vi "Read I64.vi"(7 "length":u16, 8 "error in (no error)":errorcluster, 9 "Start address":string, 10 "Read Type":variant, 11 "MelsecTCP in":refnum<class "Abs Controler.lvclass">) -> (0 "error out":errorcluster, 2 "Data":variant, 3 "MelsecTCP out":refnum<class "Abs Controler.lvclass">)   [LabVIEW 2020, in "HslCommunication.lvlib" / "Abs Controler.lvclass"]
uses:
  Abs Controler.lvclass
  E:/Git/Libraries/develop/HslCommunication/_Dependenciecs/HslCommunication.dll
  _Dependenciecs/HslCommunication.dll
  Abs Controler.lvclass/Abs Controler.ctl
  <vilib>/Utility/Data Type/NI_Data Type.lvlib
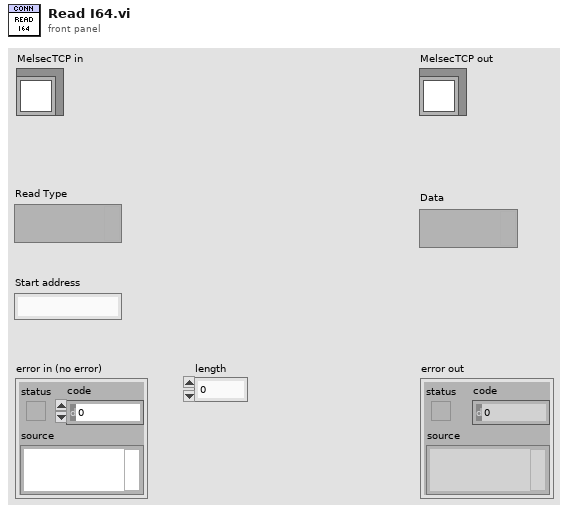
[diagram p1: front panel]
types:
  T1 = typedef "NI_Data Type.lvlib/Data Type.ctl" = enum8{"Invalid Type", "Void", "I8", "I16", "I32", "I64", "U8", "U16", "U32", "U64", "Single Float", "Double Float", "Extended Float", "Single Complex", "Double Complex", "Extended Complex", "Enum U8", "Enum U16", "Enum U32", "Enum U64", "Single Float With Unit", "Double Float With Unit", "Extended Float With Unit", "Single Complex with Unit", "Double Complex with Unit", "Extended Complex with Unit", "Boolean", "String", "Path", "Picture", "Tag", "Array", "Cluster", "Variant", "LV Variant", "Waveform", "Timestamp", "Digital Waveform", "Digital Data", "ExpressData", "Refnum", "External Data", "VI", "Poly VI", "LabVIEW Class Instance", "Fixed Point", "Set Collection", "Map Collection"}
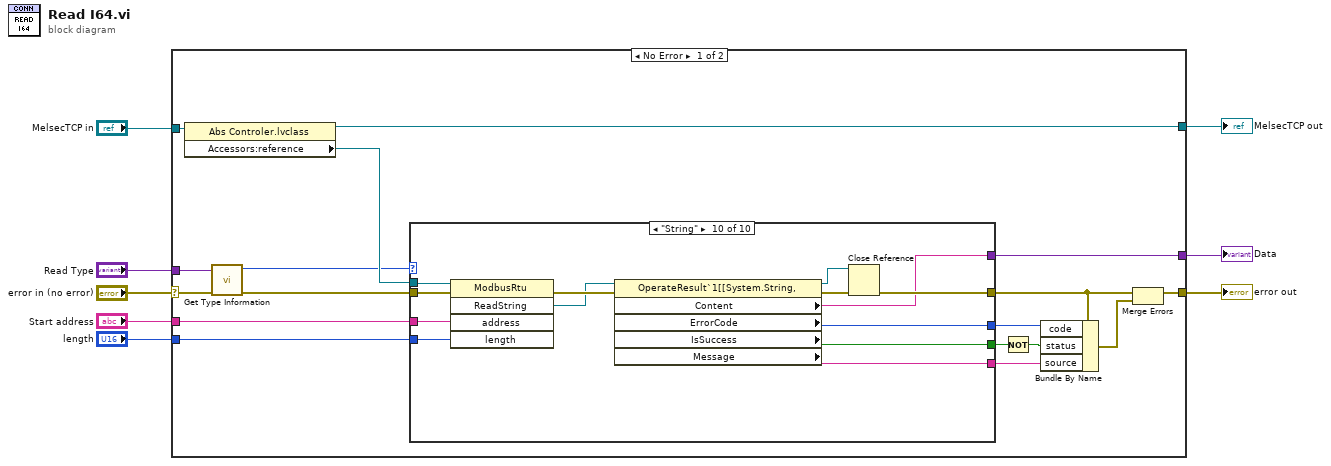
[diagram p0: block diagram]
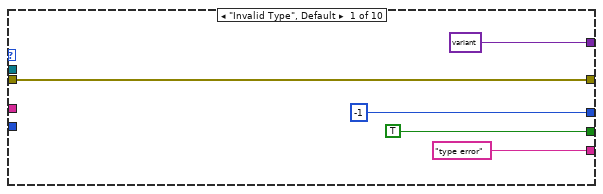
[diagram p2: hidden frame]
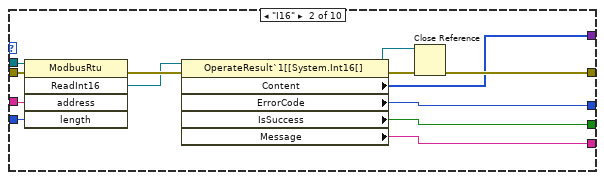
[diagram p3: hidden frame]
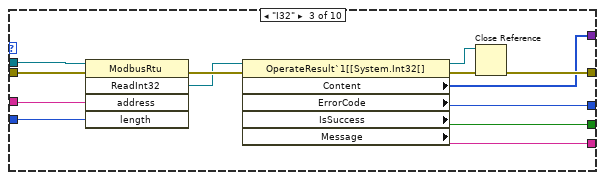
[diagram p4: hidden frame]
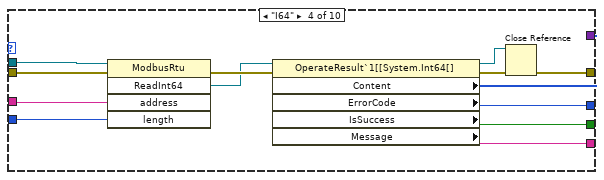
[diagram p5: hidden frame]
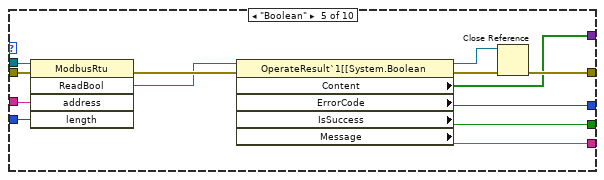
[diagram p6: hidden frame]
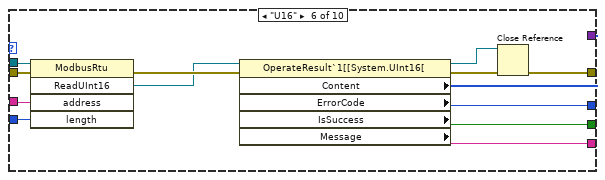
[diagram p7: hidden frame]
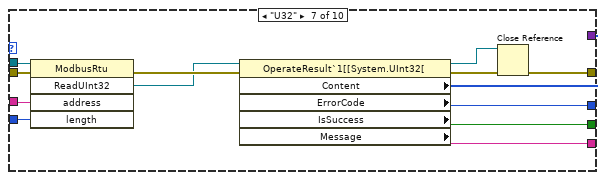
[diagram p8: hidden frame]
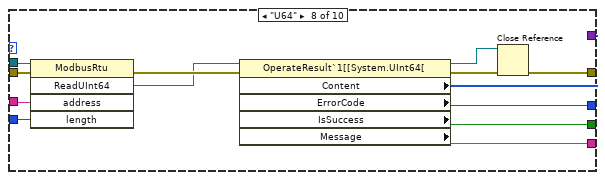
[diagram p9: hidden frame]
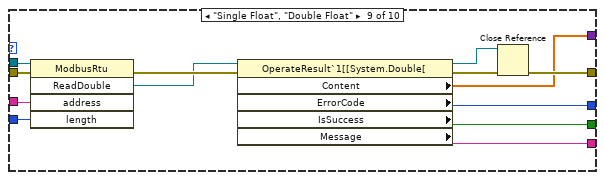
[diagram p10: hidden frame]
diagram:
  n1 = case shown="No Error" "error in (no error)" {
    selector: "error in (no error)" -> [w10 w150]
    tunnel: "MelsecTCP in" -> [w25 w149]
    tunnel: [w16 w149] -> w2
    tunnel: "Start address" -> [w13 _]
    tunnel: [w22 w150] -> w4
    tunnel: [w23 w148] -> w1
    tunnel: "length" -> [w12 _]
    tunnel: "Read Type" -> [w15 w148]
    frame No Error {
      n2 = property class="Abs Controler.lvclass"(reference=w25) -> (reference out=w16:refnum<class "Abs Controler.lvclass">, "Accessors:reference"=w24:refnum<k24>)  [unwired: 1 in, 1 out]
      n3 = call <vilib>:"Get Type Information.vi"("error in (no error)"=w10, "variant"=w15) -> ("error out"=w14:errorcluster, "type"=w11:T1)  [unwired: 5 in, 3 out]
      n4 = case shown="\"String\"" w11 {
        tunnel: w24 -> [_ w43 w56 w69 w71 w84 w97 w110 w123 w136]
        tunnel: w13 -> [_ w42 w55 w68 w82 w95 w108 w121 w134 w147]
        tunnel: w12 -> [_ w41 w54 w67 w81 w94 w107 w120 w133 w146]
        tunnel: w14 -> [w30 w40 w53 w66 w80 w93 w106 w119 w132 w145]
        tunnel: [w30 w35 w48 w61 w75 w88 w101 w114 w127 w140] -> w18
        tunnel: [variant ("Read Type") w31 w44 w57 w70 w83 w96 w109 w122 w135] -> w23
        tunnel: [-1 ("ErrorCode") w34 w47 w60 w74 w87 w100 w113 w126 w139] -> w21
        tunnel: [TRUE ("IsSuccess") w33 w46 w59 w73 w86 w99 w112 w125 w138] -> w20
        tunnel: ["type error" ("Message") w32 w45 w58 w72 w85 w98 w111 w124 w137] -> w19
        frame "Invalid Type", Default {
        }
        frame "I16" {
          n5 = invoke class="ModbusRtu" method="ReadInt16"(reference=w43, error in=w40, "address"=w42, "length"=w41) -> (error out=w39:errorcluster, "ReadInt16"=w37:refnum<k24>)  [unwired: 1 in, 3 out]
          n6 = property class="OperateResult`1[[System.Int16[]"(reference=w37, error in=w39) -> (reference out=w36:refnum<k24>, error out=w38:errorcluster, "Content"=w31:i16[], "ErrorCode"=w34:i32, "IsSuccess"=w33:bool, "Message"=w32:string)
          n7 = Close Reference(reference=w36, error in (no error)=w38) -> (error out=w35:errorcluster)
        }
        frame "I32" {
          n8 = invoke class="ModbusRtu" method="ReadInt32"(reference=w56, error in=w53, "address"=w55, "length"=w54) -> (error out=w52:errorcluster, "ReadInt32"=w50:refnum<k24>)  [unwired: 1 in, 3 out]
          n9 = property class="OperateResult`1[[System.Int32[]"(reference=w50, error in=w52) -> (reference out=w49:refnum<k24>, error out=w51:errorcluster, "Content"=w44:i32[], "ErrorCode"=w47:i32, "IsSuccess"=w46:bool, "Message"=w45:string)
          n10 = Close Reference(reference=w49, error in (no error)=w51) -> (error out=w48:errorcluster)
        }
        frame "I64" {
          n11 = invoke class="ModbusRtu" method="ReadInt64"(reference=w69, error in=w66, "address"=w68, "length"=w67) -> (error out=w65:errorcluster, "ReadInt64"=w63:refnum<k24>)  [unwired: 1 in, 3 out]
          n12 = property class="OperateResult`1[[System.Int64[]"(reference=w63, error in=w65) -> (reference out=w62:refnum<k24>, error out=w64:errorcluster, "Content"=w57:i64[], "ErrorCode"=w60:i32, "IsSuccess"=w59:bool, "Message"=w58:string)
          n13 = Close Reference(reference=w62, error in (no error)=w64) -> (error out=w61:errorcluster)
        }
        frame "Boolean" {
          n14 = invoke class="ModbusRtu" method="ReadBool"(reference=w71, error in=w80, "address"=w82, "length"=w81) -> (error out=w79:errorcluster, "ReadBool"=w77:refnum<k24>)  [unwired: 1 in, 3 out]
          n15 = property class="OperateResult`1[[System.Boolean"(reference=w77, error in=w79) -> (reference out=w76:refnum<k24>, error out=w78:errorcluster, "Content"=w70:bool[], "ErrorCode"=w74:i32, "IsSuccess"=w73:bool, "Message"=w72:string)
          n16 = Close Reference(reference=w76, error in (no error)=w78) -> (error out=w75:errorcluster)
        }
        frame "U16" {
          n17 = invoke class="ModbusRtu" method="ReadUInt16"(reference=w84, error in=w93, "address"=w95, "length"=w94) -> (error out=w92:errorcluster, "ReadUInt16"=w90:refnum<k24>)  [unwired: 1 in, 3 out]
          n18 = property class="OperateResult`1[[System.UInt16["(reference=w90, error in=w92) -> (reference out=w89:refnum<k24>, error out=w91:errorcluster, "Content"=w83:u16[], "ErrorCode"=w87:i32, "IsSuccess"=w86:bool, "Message"=w85:string)
          n19 = Close Reference(reference=w89, error in (no error)=w91) -> (error out=w88:errorcluster)
        }
        frame "U32" {
          n20 = invoke class="ModbusRtu" method="ReadUInt32"(reference=w97, error in=w106, "address"=w108, "length"=w107) -> (error out=w105:errorcluster, "ReadUInt32"=w103:refnum<k24>)  [unwired: 1 in, 3 out]
          n21 = property class="OperateResult`1[[System.UInt32["(reference=w103, error in=w105) -> (reference out=w102:refnum<k24>, error out=w104:errorcluster, "Content"=w96:u32[], "ErrorCode"=w100:i32, "IsSuccess"=w99:bool, "Message"=w98:string)
          n22 = Close Reference(reference=w102, error in (no error)=w104) -> (error out=w101:errorcluster)
        }
        frame "U64" {
          n23 = invoke class="ModbusRtu" method="ReadUInt64"(reference=w110, error in=w119, "address"=w121, "length"=w120) -> (error out=w118:errorcluster, "ReadUInt64"=w116:refnum<k24>)  [unwired: 1 in, 3 out]
          n24 = property class="OperateResult`1[[System.UInt64["(reference=w116, error in=w118) -> (reference out=w115:refnum<k24>, error out=w117:errorcluster, "Content"=w109:u64[], "ErrorCode"=w113:i32, "IsSuccess"=w112:bool, "Message"=w111:string)
          n25 = Close Reference(reference=w115, error in (no error)=w117) -> (error out=w114:errorcluster)
        }
        frame "Single Float", "Double Float" {
          n26 = invoke class="ModbusRtu" method="ReadDouble"(reference=w123, error in=w132, "address"=w134, "length"=w133) -> (error out=w131:errorcluster, "ReadDouble"=w129:refnum<k24>)  [unwired: 1 in, 3 out]
          n27 = property class="OperateResult`1[[System.Double["(reference=w129, error in=w131) -> (reference out=w128:refnum<k24>, error out=w130:errorcluster, "Content"=w122:dbl[], "ErrorCode"=w126:i32, "IsSuccess"=w125:bool, "Message"=w124:string)
          n28 = Close Reference(reference=w128, error in (no error)=w130) -> (error out=w127:errorcluster)
        }
        frame "String" {
          n29 = invoke class="ModbusRtu" method="ReadString"(reference=w136, error in=w145, "address"=w147, "length"=w146) -> (error out=w144:errorcluster, "ReadString"=w142:refnum<k24>)  [unwired: 1 in, 3 out]
          n30 = property class="OperateResult`1[[System.String,"(reference=w142, error in=w144) -> (reference out=w141:refnum<k24>, error out=w143:errorcluster, "Content"=w135:string, "ErrorCode"=w139:i32, "IsSuccess"=w138:bool, "Message"=w137:string)
          n31 = Close Reference(reference=w141, error in (no error)=w143) -> (error out=w140:errorcluster)
        }
      }
      n32 = Not(x=w20) -> (.not. x?=w9:bool)
      n33 = Bundle By Name(cluster=w18, "code"=w21, "status"=w9, "source"=w19) -> (w17:errorcluster)
      n34 = Merge Errors(w18, w17) -> (w22:errorcluster)
    }
    frame Error {
    }
  }
  "error out" <- w4
  "MelsecTCP out" <- w2
  "Data" <- w1
